vi "GetStructureReference.vi"(8 "error in":errorcluster, 11 "Structure in":refnum<class "Structure.lvclass">) -> (0 "error out":errorcluster, 1 "reference out":refnum<vi>, 3 "Structure out":refnum<class "Structure.lvclass">)   [LabVIEW 2014, in "Structure.lvclass"]
uses:
  Structure.lvclass
  Generic/Generic.lvclass
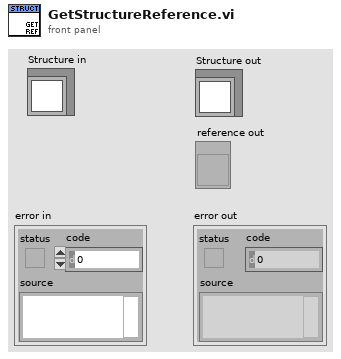
[diagram p1: front panel]
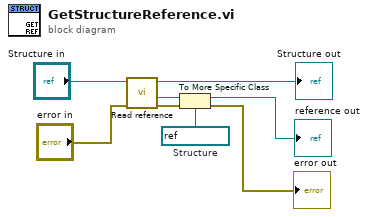
[diagram p0: block diagram]
diagram:
  w5 = refnum<vi> refnum  # Structure
  n1 = call "Read reference.vi"("error in"="error in", "GObject in"="Structure in") -> ("error out"=w6:errorcluster, "reference"=w7:refnum<vi>, "GObject out"=→"Structure out":refnum<class "Structure.lvclass">)  [unwired: 5 in]
  n2 = To More Specific Class(target class=w5, reference=w7, error in=w6) -> (specific class reference=→"reference out":refnum<vi>, error out=→"error out":errorcluster)
